vi "Cleanup.vi"(6 "Queue Name":string="firmata-serial-communication", 8 "error in":errorcluster) -> (0 "error out":errorcluster)   [LabVIEW 2020, in "FirmataClient.lvlib"]
doc: "Cleanup the library references, data and the actively selected transport (i.e. serial comport)"
uses:
  FirmataClient.lvlib
  Transports/Controls/Transport Commands.ctl
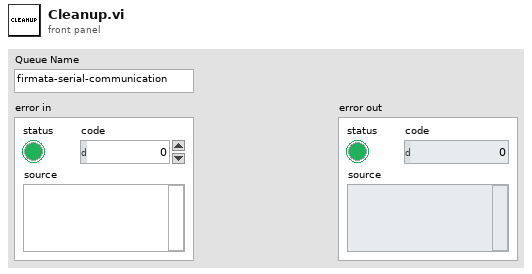
[diagram p1: front panel]
types:
  T1 = typedef "Transport Commands.ctl" = enum16{"Initialize", "Transmit - Receive", "Cleanup", "Cleanup And Stop"}
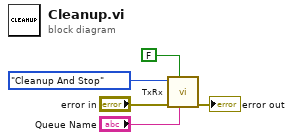
[diagram p0: block diagram]
diagram:
  n1 = call "TxRx.vi"("Queue Name"="Queue Name", "Wait For Reply?"=FALSE, "error in"="error in", "Command"=Transport_Commands."Cleanup And Stop") -> ("error out"=→"error out":errorcluster)  [unwired: 6 in, 1 out]
